vi "Compass Parser.vi"(8 "error in (no error)":errorcluster, 10 "RDS Serial Frame":refnum<class "RDS Serial Frame.lvclass">, 11 "Compass Instrument in":refnum<class "Compass Instrument.lvclass">) -> (0 "error out":errorcluster, 2 "RDS Message out":refnum<class "Compass Data Message.lvclass">, 3 "Compass Instrument out":refnum<class "Compass Instrument.lvclass">)   [LabVIEW 2015, in "Compass Instrument.lvlib" / "Compass Instrument.lvclass"]
uses:
  Compass Instrument.lvclass
  MCB Instrument/MCB Instrument/MCB Instrument.lvclass
  RDS Framework/RDS Message Class/RDS Message.lvclass
  RDS Serial Handler/RDS Serial Frame.lvclass
  RDS Child Messages/Compass/Compass Data Message.lvclass
  RDS Serial Handler/RDS Serial Frame.lvclass/RDS Serial Frame.ctl
  RDS Framework/RDS Message ID.ctl
  Compass Instrument.lvclass/Compass Instrument.ctl
  RDS Child Messages/Compass/Compass Data Message.lvclass/Compass Data Message.ctl
  RDS Framework/RDS Message Class/RDS Message.lvclass/RDS Message.ctl
  RDS Serial Handler/RDS Serial Handler.lvlib
  RDS Child Messages/RDS Child Messages.lvlib
  RDS Child Messages/MCB/MCB Status Message/MCB Status.lvclass
  RDS Child Messages/MCB/MCB Motor Status.ctl
panel:
  in  "RDS Serial Frame":refnum<class "RDS Serial Frame.lvclass">
  out "RDS Framework.lvlib:RDS Message.lvclass":refnum<class "RDS Message.lvclass">
  out "MCB Instrument out":refnum<class "MCB Instrument.lvclass">
  in  "MCB Instrument in":refnum<class "MCB Instrument.lvclass">
  in  "error in (no error) 2":errorcluster
  out "error out 2":errorcluster
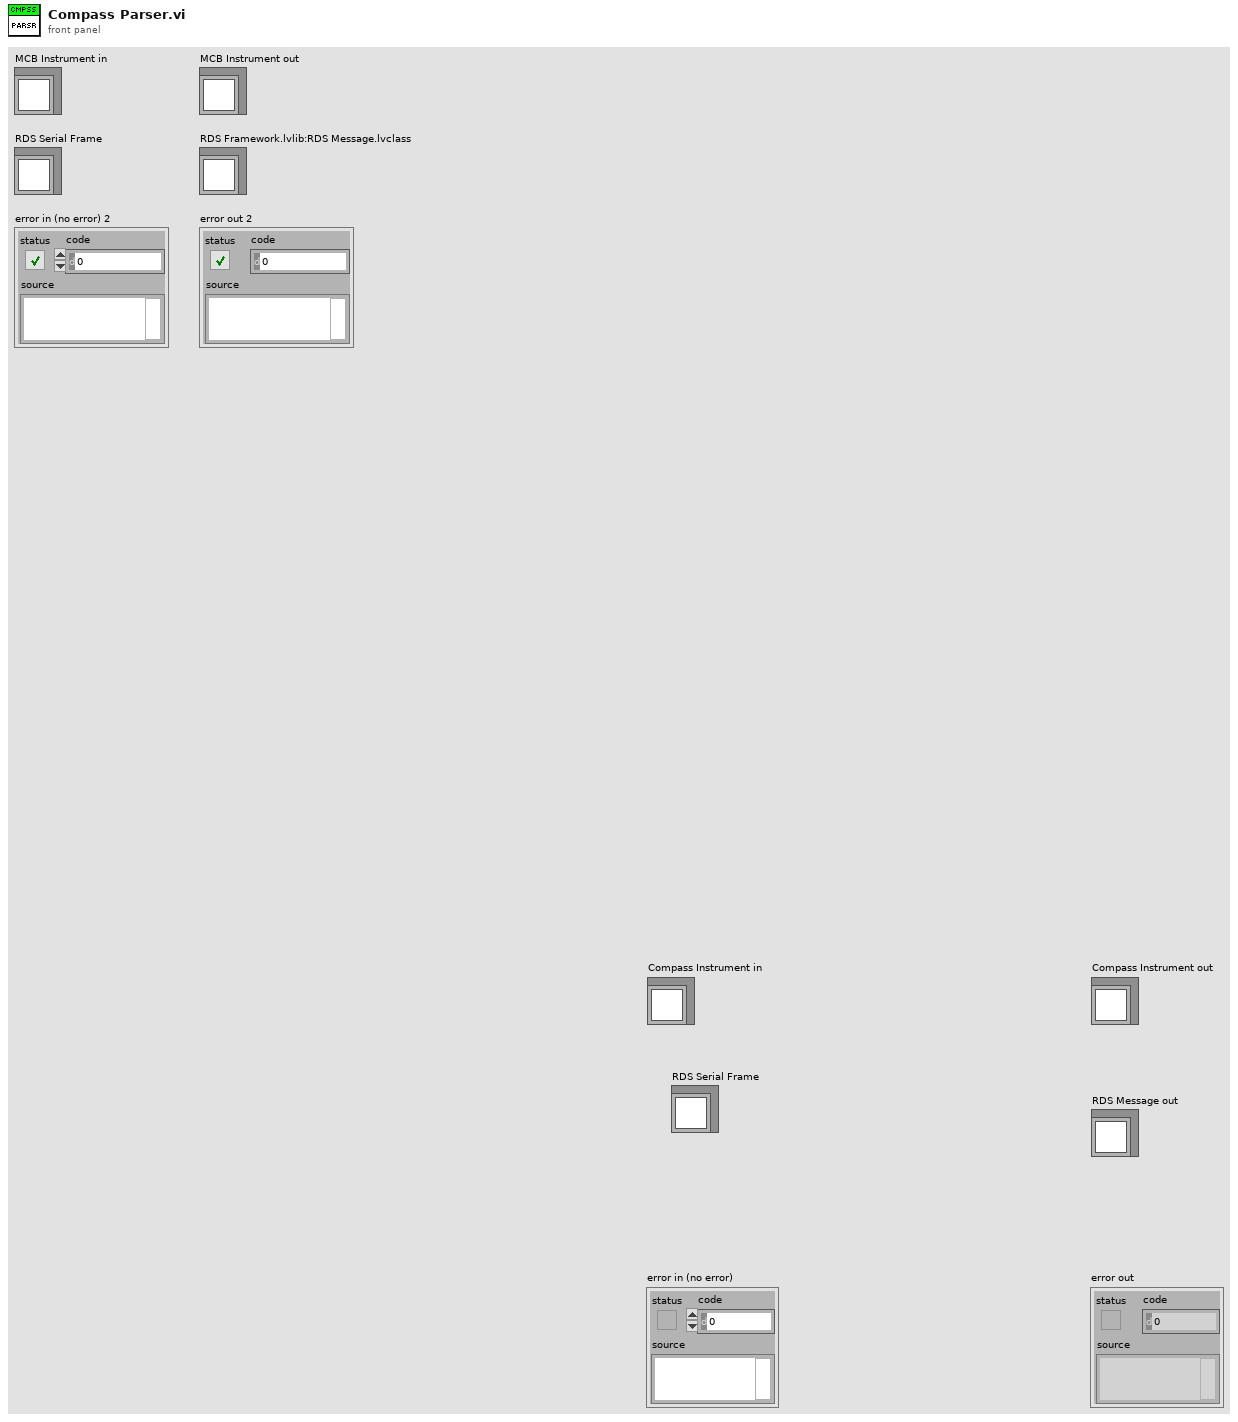
[diagram p1: front panel]
types:
  T1 = typedef "RDS Child Messages.lvlib/RDS Message ID.ctl" = enum16{"RDS Hello World", "String Message", "AIP_Status", "AIP_Command", "GPS_Data", "MCB_Command", "MCB_Status", "Compass_Data", "Depth_Data", "Battery_Data", "Contoller_State", "Set_Mag_Dev", "BTB_Shutdown", "State_Sample_Request", "State_Sample", "PID_Gains_Set", "Helm_Limiter_Set", "Helm_Heading_Command", "Helm_Steering_Command", "Helm_Status", "Controller_Message", "AIP_Set_Min_Depth", "Mission_Controller_State", "Mission_Upload", "Mission_Set_Op_and_Run", "Mission_Settings_Set"}
  T2 = typedef "RDS Child Messages.lvlib/MCB Motor Status.ctl" = cluster{"Motor Power":i16, "Motor Command":i16, "Battery Volts":sgl, "Battery Amps":sgl, "Motor Amps":sgl, "MCU Temp":i16, "Heatsink Temp":i16, "Fault Flags":u16, "StatusFlags":u16}
  T3 = typedef "RDS Instrument Library.lvlib/Compass Data.ctl" = cluster{"Compass Heading":sgl, "pitch Angle":sgl, "roll Angle":sgl, "Temperature":sgl, "Depth":sgl, "Magnetic Field":sgl, "Magnetic Field X":sgl, "Magnetic Field Y":sgl, "Magnetic Field Z":sgl, "Acceleration":sgl, "Acceleration X":sgl, "Acceleration Y":sgl, "Gyro":sgl, "Gyro X":sgl, "Acceleration Z":sgl, "Gyro Y":sgl, "Raw Heading":sgl}
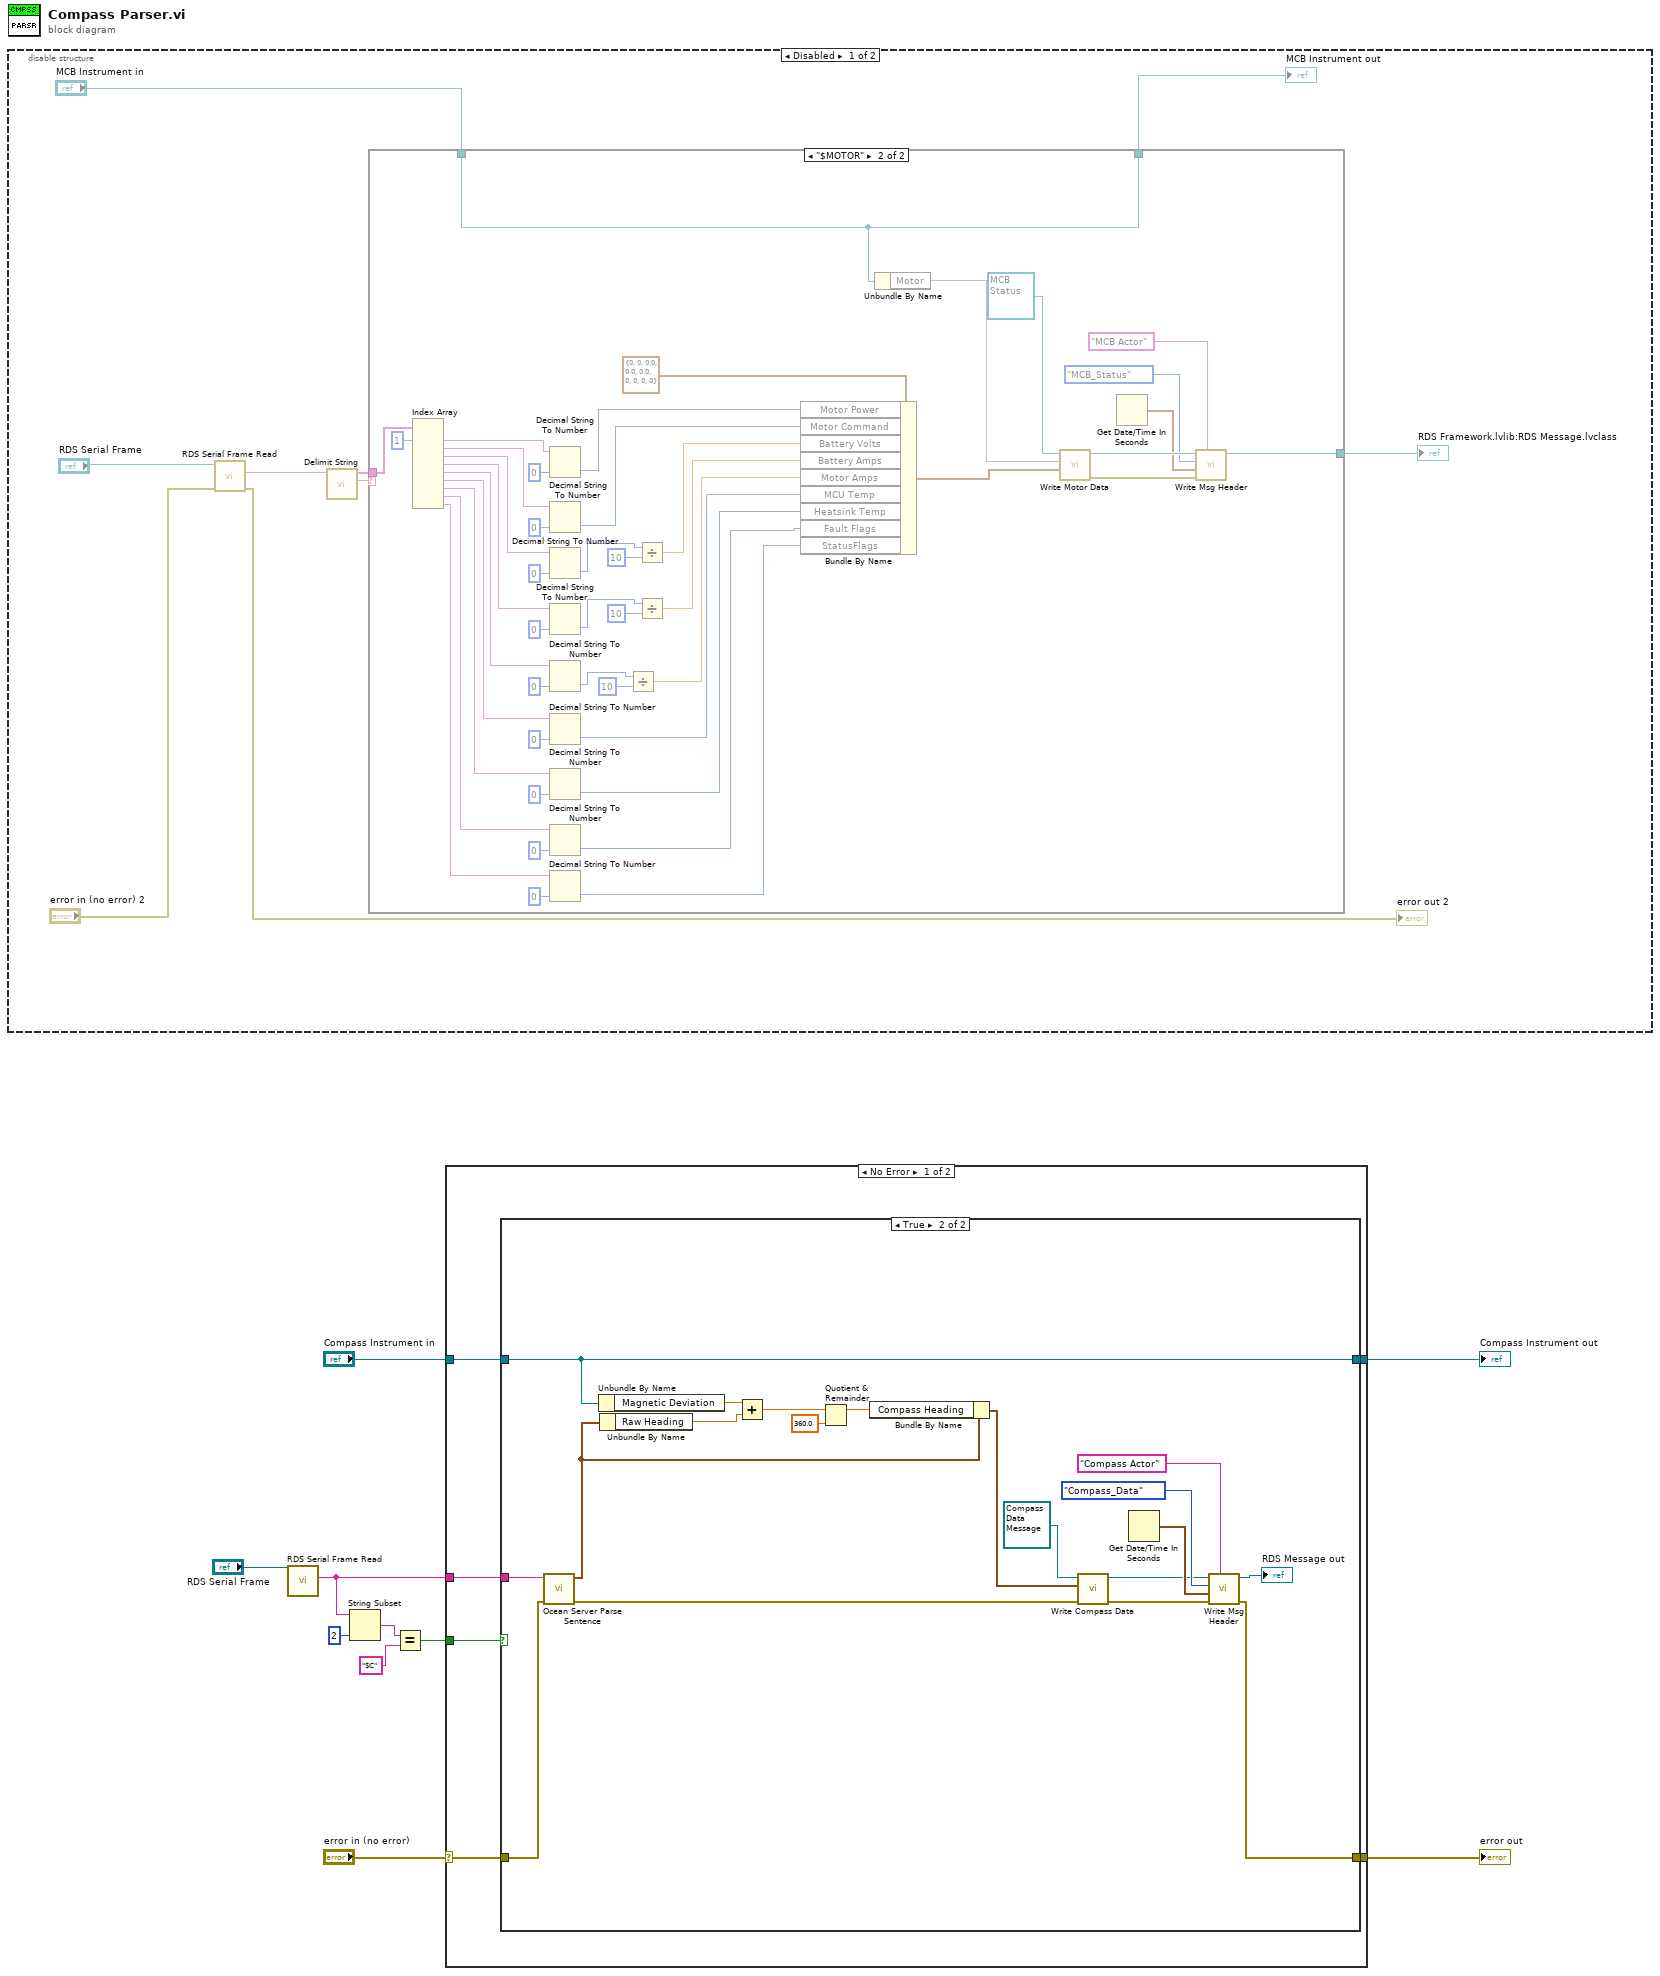
[diagram p0: block diagram]
diagram:
  n1 = disable-structure shown="Disabled" {
    frame Disabled {
      n2 = call "RDS Serial Frame Read.vi"("error in (no error)"="error in (no error) 2", "RDS Serial Frame in"="RDS Serial Frame") -> ("error out"=→"error out 2":errorcluster, "Serial String"=w13:string)  [unwired: 6 in, 2 out]
      n3 = call "Delimit String.vi"("Serial String"=w13) -> ("First Element"=w14:string, "All Elements"=w15:string[])  [unwired: 9 in]
      n4 = case shown="\"$MOTOR\"" w14 {
        tunnel: w15 -> [_ w65]
        tunnel: [w20 w63] -> w16
        tunnel: "MCB Instrument in" -> [w20 w63]
        tunnel: [_ w31] -> w11
        frame "False", Default {
        }
        frame "$MOTOR" {
          n5 = Index Array(array=w65, index #1=1 ("index")) -> (element #1=w64:string, element #2=w60:string, element #3=w56:string, element #4=w49:string, element #5=w46:string, element #6=w43:string, element #7=w41:string, element #8=w40:string, element #9=w22:string)  [unwired: 8 in]
          n6 = Decimal String To Number(string=w64, default (0L)=i16 0 ("default (0 I32)")) -> (number=w62:i16)  [unwired: 1 in, 1 out]
          n7 = Decimal String To Number(string=w60, default (0L)=i16 0 ("default (0 I32)")) -> (number=w59:i16)  [unwired: 1 in, 1 out]
          n8 = Decimal String To Number(string=w56, default (0L)=i16 0 ("default (0 I32)")) -> (number=w55:i16)  [unwired: 1 in, 1 out]
          n9 = Decimal String To Number(string=w49, default (0L)=i16 0 ("default (0 I32)")) -> (number=w51:i16)  [unwired: 1 in, 1 out]
          n10 = Decimal String To Number(string=w46, default (0L)=i16 0 ("default (0 I32)")) -> (number=w29:i16)  [unwired: 1 in, 1 out]
          n11 = Decimal String To Number(string=w43, default (0L)=i16 0 ("default (0 I32)")) -> (number=w27:i16)  [unwired: 1 in, 1 out]
          n12 = Decimal String To Number(string=w41, default (0L)=u16 0 ("default (0 I32)")) -> (number=w26:u16)  [unwired: 1 in, 1 out]
          n13 = Decimal String To Number(string=w40, default (0L)=u16 0 ("default (0 I32)")) -> (number=w25:u16)  [unwired: 1 in, 1 out]
          n14 = Decimal String To Number(string=w22, default (0L)=u16 0 ("default (0 I32)")) -> (number=w21:u16)  [unwired: 1 in, 1 out]
          n15 = Divide(x=w29, y=i16 10) -> (x/y=w28:dbl)
          n16 = Divide(x=w55, y=i16 10) -> (x/y=w53:dbl)
          n17 = Divide(x=w51, y=i16 10) -> (x/y=w48:dbl)
          n18 = Bundle By Name(cluster=T2 {"Motor Power"=0, "Motor Command"=0, "Battery Volts"=0.0, "Battery Amps"=0.0, "Motor Amps"=0.0, "MCU Temp"=0, "Heatsink Temp"=0, "Fault Flags"=0, "StatusFlags"=0} ("Motor Data"), "Motor Power"=w62, "Motor Command"=w59, "Battery Volts"=w53, "Battery Amps"=w48, "Motor Amps"=w28, "MCU Temp"=w27, "Heatsink Temp"=w26, "Fault Flags"=w25, "StatusFlags"=w21) -> (w37:T2)
          n19 = Unbundle By Name(w63) -> ("Motor"=w38)
          n20 = call "Write Motor Data.vi"("Motor Data"=w37, "Motor"=w38, "MCB Status in"=refnum<class "MCB Status.lvclass"> refnum) -> ("error out"=w32:errorcluster, "MCB Status out"=w36:refnum<class "MCB Status.lvclass">)  [unwired: 7 in]
          n21 = Get Date/Time In Seconds() -> (seconds since 1Jan1904=w33:timestamp)
          n22 = call "Write Msg Header.vi"("Sender Name"="MCB Actor", "error in (no error)"=w32, "Time Stamp"=w33, "Msg ID"=RDS_Message_ID."MCB_Status", "RDS Message in"=w36) -> ("RDS Message out"=w31:refnum<class "MCB Status.lvclass">)  [unwired: 5 in, 1 out]
        }
      }
      "MCB Instrument out" <- w16
      "RDS Framework.lvlib:RDS Message.lvclass" <- w11
    }
    frame Enabled {
    }
  }
  n23 = call "RDS Serial Frame Read.vi"("RDS Serial Frame in"="RDS Serial Frame") -> ("Serial String"=w1:string)  [unwired: 7 in, 3 out]
  n24 = String Subset(string=w1, length (rest)=2 ("length (rest)")) -> (substring=w4:string)  [unwired: 1 in]
  n25 = Equal?(x=w4, y="$C") -> (x = y?=w2:bool)
  n26 = case shown="No Error" "error in (no error)" {
    selector: "error in (no error)" -> [w69 w95]
    tunnel: [w70 w95] -> w9
    tunnel: [w72 w94] -> w7
    tunnel: "Compass Instrument in" -> [w71 w94]
    tunnel: w2 -> [w68 _]
    tunnel: w1 -> [w67 _]
    frame No Error {
      n27 = case shown="True" w68 {
        tunnel: [w74 w81] -> w72
        tunnel: w71 -> [w74 w81]
        tunnel: [w73 w83] -> w70
        tunnel: w69 -> [w73 w84]
        tunnel: w67 -> [_ w93]
        frame False {
        }
        frame True {
          n28 = call "Ocean Server Parse Sentence.vi"("error in (no error)"=w84, "Ocean Server Sentence"=w93) -> ("error out"=w85:errorcluster, "Values"=w82:T3)  [unwired: 8 in]
          n29 = Unbundle By Name(w81) -> ("Magnetic Deviation"=w79:sgl)
          n30 = Unbundle By Name(w82) -> ("Raw Heading"=w80:sgl)
          n31 = Add(x=w79, y=w80) -> (x+y=w76:sgl)
          n32 = Quotient & Remainder(x=w76, y=sgl 360.0) -> (x-y*floor(x/y)=w75:sgl)  [unwired: 1 out]
          n33 = Bundle By Name(cluster=w82, "Compass Heading"=w75) -> (w78:T3)
          n34 = call "Write Compass Data.vi"("error in (no error)"=w85, "Compass Data"=w78, "Compass Data Message in"=refnum<class "Compass Data Message.lvclass"> refnum ("RDS Child Messages.lvlib:Compass Data Message.lvclass")) -> ("error out"=w87:errorcluster, "Compass Data Message out"=w88:refnum<class "Compass Data Message.lvclass">)  [unwired: 7 in]
          n35 = Get Date/Time In Seconds() -> (seconds since 1Jan1904=w89:timestamp)
          n36 = call "Write Msg Header.vi"("Sender Name"="Compass Actor", "error in (no error)"=w87, "Time Stamp"=w89, "Msg ID"=RDS_Message_ID."Compass_Data", "RDS Message in"=w88) -> ("error out"=w83:errorcluster, "RDS Message out"=→"RDS Message out":refnum<class "Compass Data Message.lvclass">)  [unwired: 5 in]
        }
      }
    }
    frame Error {
    }
  }
  "error out" <- w9
  "Compass Instrument out" <- w7
